vi "create.authorization_header.vi"(6 "Content Type":string="application/json", 8 "error in":errorcluster, 10 "specific headers in":cluster{"header":string, "value":string}[](array[cluster]), 11 "Nominal Client in":refnum<class "Nominal Client.lvclass">) -> (0 "error out":errorcluster, 2 "specific headers out":cluster{"header":string, "value":string}[](array[cluster]), 3 "Nominal Client out":refnum<class "Nominal Client.lvclass">)   [LabVIEW 2020, in "Nominal Client.lvclass"]
uses:
  Nominal Client.lvclass
  Nominal Client.lvclass/Nominal Client.ctl
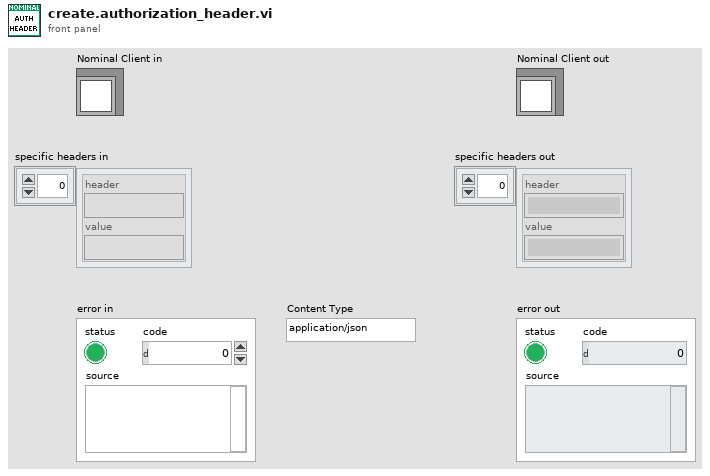
[diagram p1: front panel]
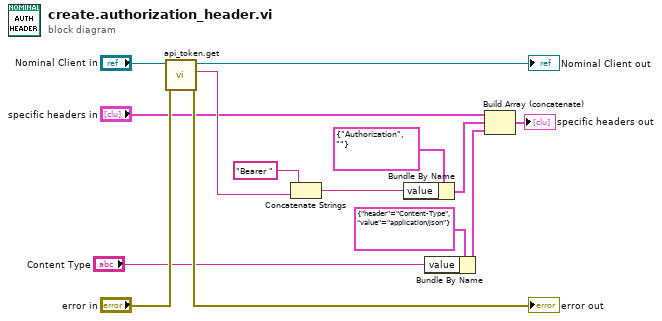
[diagram p0: block diagram]
diagram:
  n1 = call "api_token.get.vi"("error in"="error in", "Nominal Client in"="Nominal Client in") -> ("error out"=→"error out":errorcluster, "API Token"=w9:string, "Nominal Client out"=→"Nominal Client out":refnum<class "Nominal Client.lvclass">)  [unwired: 7 in]
  n2 = Concatenate Strings("Bearer " ("value"), w9) -> (w10:string)
  n3 = Bundle By Name(cluster=cluster{"header":string, "value":string} {"header"="Authorization", "value"=""} ("Header"), "value"=w10) -> (w8:cluster{"header":string, "value":string})
  n4 = Bundle By Name(cluster=cluster{"header":string, "value":string} {"header"="Content-Type", "value"="application/json"} ("Header"), "value"="Content Type") -> (w1:cluster{"header":string, "value":string})
  n5 = Build Array (concatenate)("specific headers in", w8, w1) -> (→"specific headers out":cluster{"header":string, "value":string}[])
